vi "CSDB_Config.set Names.vi"(2 "Name":string) -> (16 "Names":string[](array[string]))   [LabVIEW 2014, in "CSDB_Config.lvlib"]
doc: "Constructs names for, as an example, instances to be added"
uses:
  CSDB_Config.lvlib
panel:
  in  "Multicolumn Listbox":i32(listbox)
  in  "ADD an INDEX":enum32{"numerical", "alphabetical"}(tab)
  in  "starting number":dbl
  in  "starting letter":string
  in  "clear":bool
  in  "stop":bool
  in  "#":i32=1 min=1
  in  "suf":bool
  in  "pref":bool
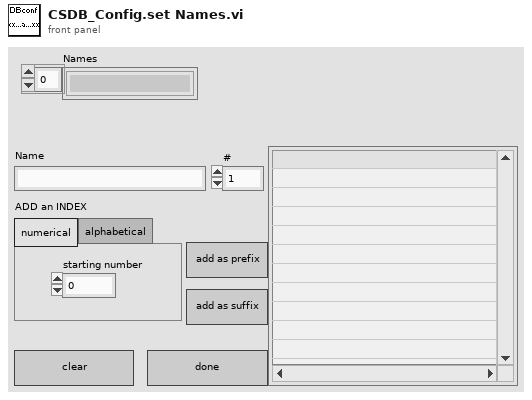
[diagram p1: front panel]
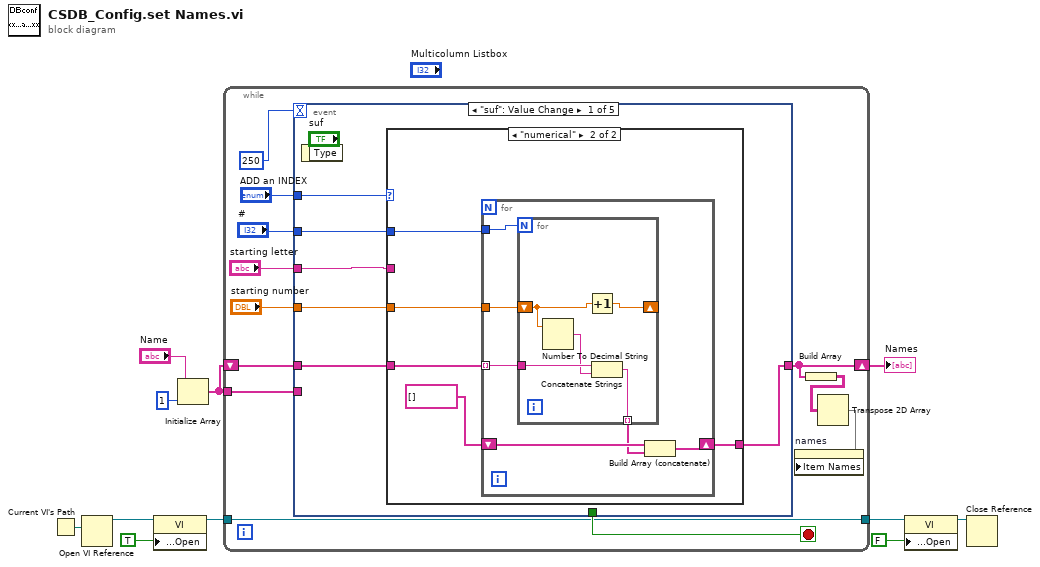
[diagram p0: block diagram]
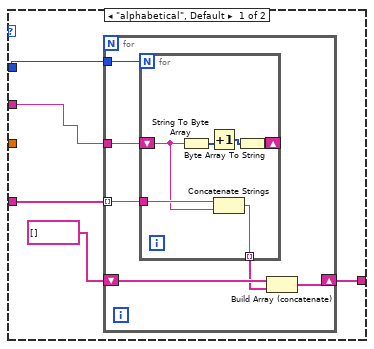
[diagram p2: hidden frame]
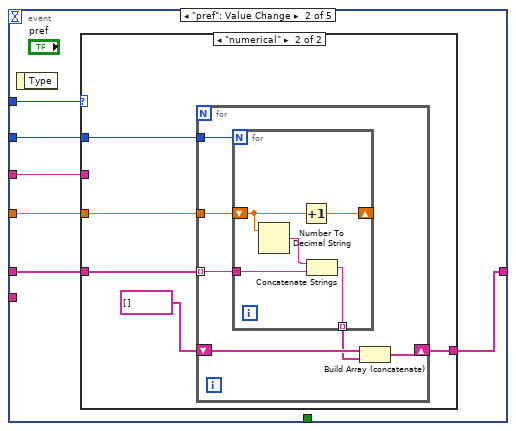
[diagram p3: hidden frame]
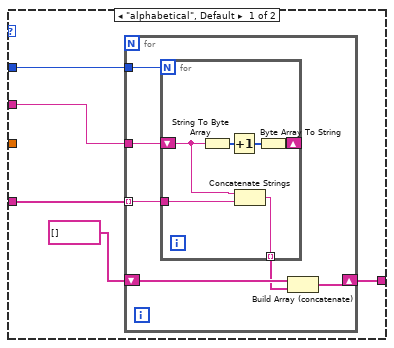
[diagram p4: hidden frame]
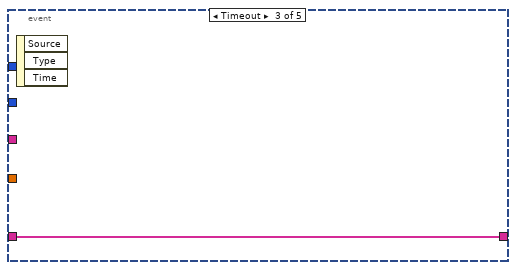
[diagram p5: hidden frame]
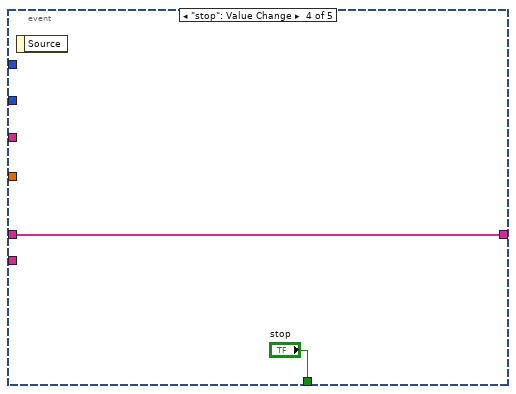
[diagram p6: hidden frame]
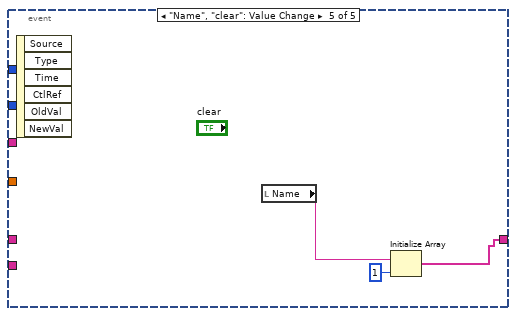
[diagram p7: hidden frame]
diagram:
  n1 = Current VI's Path() -> (path=w8:path)
  n2 = Open VI Reference(vi path=w8) -> (vi reference=w7:refnum<vi>)  [unwired: 5 in, 1 out]
  n3 = property class="VI"(reference=w7, "Front Panel Window:Open"=TRUE) -> (reference out=w5:refnum<vi>)  [unwired: 1 in, 1 out]
  n4 = Initialize Array("Name", 1 ("dimension size")) -> (w9:string[])
  n5 = while {
    shift-right: [w14] -> w1
    shift-left: w9 -> [w23]
    tunnel: w9 -> [w20]
    tunnel: [w19] -> w3
    tunnel: w5 -> [w19]
    stop <- w22 stop-if-true
    n6 = event shown="[0] \"suf\": Value Change" {
      selector: _ -> [_ _ _ _ _]
      dyn-events: _ -> [_ _ _ _ _]
      timeout: 250 -> [_ _ _ _ _]
      tunnel: w23 -> [w29 w68 w102 w103 _]
      tunnel: [w28 w67 w102 w103 w105] -> w14
      tunnel: [_ _ _ "stop" _] -> w22
      tunnel: "#" -> [w25 w66 _ _ _]
      tunnel: "starting letter" -> [w24 w65 _ _ _]
      tunnel: w20 -> [_ _ _ _ _]
      tunnel: "ADD an INDEX" -> [w26 w64 _ _ _]
      tunnel: "starting number" -> [w27 w63 _ _ _]
      event "suf": Value Change {
        n7 = event-data() -> ()  [unwired: 1 in, 1 out]
        n8 = case shown="\"numerical\"" w26 {
          tunnel: w29 -> [w34 w51]
          tunnel: [w32 w49] -> w28
          tunnel: w25 -> [w31 w48]
          tunnel: w24 -> [w30 _]
          tunnel: w27 -> [_ w47]
          frame "alphabetical", Default {
            n9 = for {
              tunnel: w34 -> [w40] mode=indexing
              tunnel: w31 -> [w39]
              tunnel: w30 -> [w38]
              shift-right: [w35] -> w32
              shift-left: string[] [] ("Array 2") -> [w37]
              n10 = for {
                N: w39 -> [_]
                tunnel: w40 -> [w46]
                shift-right: [w43] -> _
                shift-left: w38 -> [w42]
                tunnel: [w41] -> w36 mode=indexing
                n11 = String To Byte Array(string=w42) -> (unsigned byte array=w44:u8[])
                n12 = Increment(x=w44) -> (x+1=w45:u8[])
                n13 = Concatenate Strings(w46, w42) -> (w41:string)
                n14 = Byte Array To String(unsigned byte array=w45) -> (string=w43:string)
              }
              n15 = Build Array (concatenate)(w37, w36) -> (w35:string[])
            }
          }
          frame "numerical" {
            n16 = for {
              tunnel: w51 -> [w57] mode=indexing
              tunnel: w48 -> [w56]
              tunnel: w47 -> [w55]
              shift-right: [w52] -> w49
              shift-left: string[] [] ("Array 2") -> [w54]
              n17 = for {
                N: w56 -> [_]
                tunnel: w57 -> [w62]
                shift-right: [w60] -> _
                shift-left: w55 -> [w59]
                tunnel: [w61] -> w53 mode=indexing
                n18 = Number To Decimal String(number=w59) -> (decimal integer string=w58:string)  [unwired: 1 in]
                n19 = Increment(x=w59) -> (x+1=w60:dbl)
                n20 = Concatenate Strings(w62, w58) -> (w61:string)
              }
              n21 = Build Array (concatenate)(w54, w53) -> (w52:string[])
            }
          }
        }
      }
      event "pref": Value Change {
        n22 = event-data() -> ()  [unwired: 1 in, 1 out]
        n23 = case shown="\"numerical\"" w64 {
          tunnel: w68 -> [w73 w90]
          tunnel: [w71 w88] -> w67
          tunnel: w66 -> [w70 w87]
          tunnel: w65 -> [w69 _]
          tunnel: w63 -> [_ w86]
          frame "alphabetical", Default {
            n24 = for {
              tunnel: w73 -> [w79] mode=indexing
              tunnel: w70 -> [w78]
              tunnel: w69 -> [w77]
              shift-right: [w74] -> w71
              shift-left: string[] [] ("Array 2") -> [w76]
              n25 = for {
                N: w78 -> [_]
                tunnel: w79 -> [w85]
                shift-right: [w82] -> _
                shift-left: w77 -> [w80]
                tunnel: [w81] -> w75 mode=indexing
                n26 = String To Byte Array(string=w80) -> (unsigned byte array=w83:u8[])
                n27 = Increment(x=w83) -> (x+1=w84:u8[])
                n28 = Concatenate Strings(w80, w85) -> (w81:string)
                n29 = Byte Array To String(unsigned byte array=w84) -> (string=w82:string)
              }
              n30 = Build Array (concatenate)(w76, w75) -> (w74:string[])
            }
          }
          frame "numerical" {
            n31 = for {
              tunnel: w90 -> [w96] mode=indexing
              tunnel: w87 -> [w95]
              tunnel: w86 -> [w94]
              shift-right: [w91] -> w88
              shift-left: string[] [] ("Array 2") -> [w93]
              n32 = for {
                N: w95 -> [_]
                tunnel: w96 -> [w101]
                shift-right: [w99] -> _
                shift-left: w94 -> [w98]
                tunnel: [w100] -> w92 mode=indexing
                n33 = Number To Decimal String(number=w98) -> (decimal integer string=w97:string)  [unwired: 1 in]
                n34 = Increment(x=w98) -> (x+1=w99:dbl)
                n35 = Concatenate Strings(w97, w101) -> (w100:string)
              }
              n36 = Build Array (concatenate)(w93, w92) -> (w91:string[])
            }
          }
        }
      }
      event Timeout {
        n37 = event-data() -> ()  [unwired: 1 in, 3 out]
      }
      event "stop": Value Change {
        n38 = event-data() -> ()  [unwired: 1 in, 1 out]
      }
      event "Name", "clear": Value Change {
        n39 = event-data() -> ()  [unwired: 1 in, 6 out]
        n40 = local read "Name"() -> (w106:string)
        n41 = Initialize Array(w106, 1 ("dimension size")) -> (w105:string[])
      }
    }
    n42 = Build Array(w14) -> (w13:string[][])
    n43 = Transpose 2D Array(2D array=w13) -> (transposed array=w12:string[][])
    n44 = property on="names" class="MCListbox (strict)"("Item Names"=w12) -> ()  [unwired: 2 in, 2 out]
  }
  "Names" <- w1
  n45 = property class="VI"(reference=w3, "Front Panel Window:Open"=FALSE) -> (reference out=w2:refnum<vi>)  [unwired: 1 in, 1 out]
  n46 = Close Reference(reference=w2) -> ()  [unwired: 1 in, 1 out]
